vi "3-9 warnings with wind speed.vi"() -> ()   [LabVIEW 2015]
doc: "This simple VI thorws a warning if the Current temp input is greater than the max temp input or less than the min temp input."
panel:
  in  "Current Wind Speed":dbl
  in  "Max Wind Speed":dbl
  out "Warning?":bool
  out "Warning Text":string
  in  "Max Temp":dbl=30.0
  in  "Min Temp":dbl=10.0
  in  "Current Temp":dbl=25.0
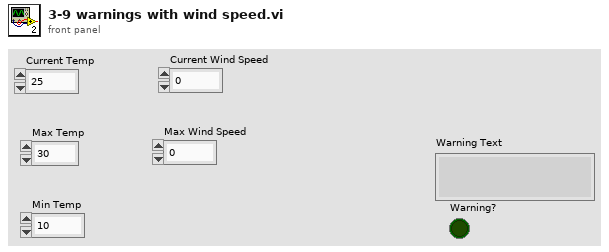
[diagram p1: front panel]
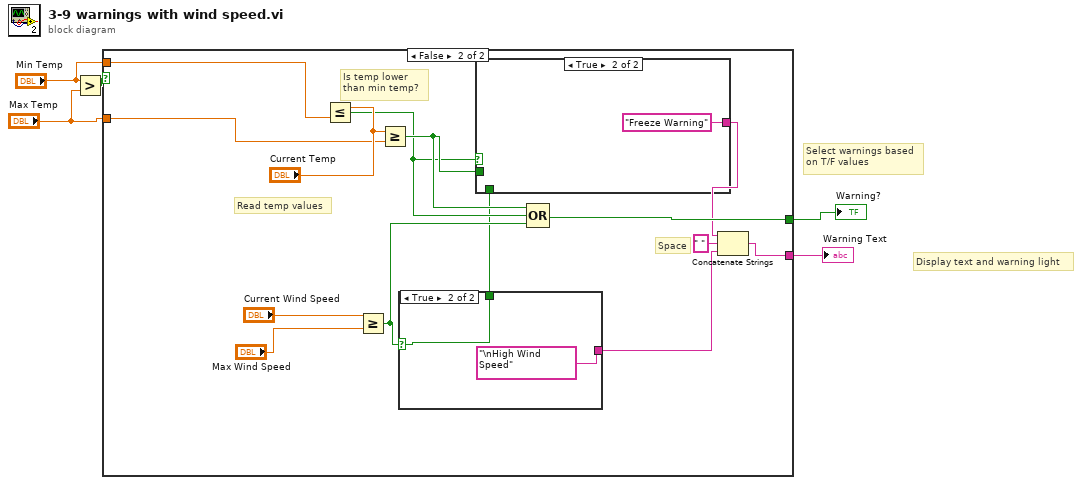
[diagram p0: block diagram]
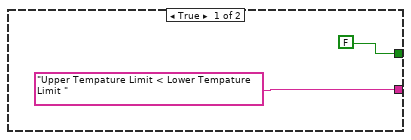
[diagram p2: hidden frame]
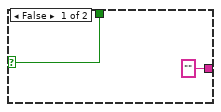
[diagram p3: hidden frame]
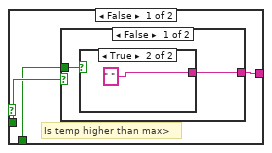
[diagram p4: hidden frame]
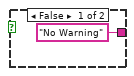
[diagram p5: hidden frame]
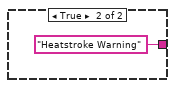
[diagram p6: hidden frame]
diagram:
  # "Display text and warning light"
  # "Select warnings based\non T/F values"
  n1 = Greater?(x="Min Temp", y="Max Temp") -> (0:w4:bool)
  n2 = case shown="False" w4 {
    tunnel: "Max Temp" -> [_ w20]
    tunnel: "Min Temp" -> [_ w19]
    tunnel: [FALSE w18] -> w5
    tunnel: ["Upper Tempature Limit < Lower Tempature Limit " w11] -> w1
    frame True {
    }
    frame False {
      # "Space"
      # "Read temp values"
      # "Is temp lower \nthan min temp?"
      n3 = Less Or Equal?(x="Current Temp", y=w19) -> (x <= y?=w9:bool)
      n4 = Greater Or Equal?(x="Current Wind Speed", y="Max Wind Speed") -> (x >= y?=w15:bool)
      n5 = Greater Or Equal?(x="Current Temp", y=w20) -> (x >= y?=w10:bool)
      n6 = case shown="True" w15 {
        selector: w15 -> [w22 w24]
        tunnel: ["" "\nHigh Wind Speed"] -> w13
        tunnel: [w22 w24] -> w8
        frame False {
        }
        frame True {
        }
      }
      n7 = case shown="True" w9 {
        tunnel: [w27 "Freeze Warning"] -> w12
        tunnel: w10 -> [w28 _]
        tunnel: w8 -> [w26 _]
        frame False {
          # "Is temp higher than max>"
          n8 = case shown="False" w28 {
            tunnel: [w30 "Heatstroke Warning"] -> w27
            tunnel: w26 -> [w29 _]
            frame False {
              n9 = case shown="True" w29 {
                tunnel: ["No Warning" " "] -> w30
                frame False {
                }
                frame True {
                }
              }
            }
            frame True {
            }
          }
        }
        frame True {
        }
      }
      n10 = Compound Arithmetic op=OR(w10, w9, w15) -> (w18:bool)
      n11 = Concatenate Strings(w12, " " ("string"), w13) -> (w11:string)
    }
  }
  "Warning Text" <- w1
  "Warning?" <- w5
